vi "IMU Correction.vi"(6 "Enable IMU":bool, 8 "Current Angle":dbl, 9 "Desired Angle (Relative)":dbl, 10 "Iterations":dbl, 11 "PID gains":T1 {"derivative time (Td, min)" format="%.3f"; "integral time (Ti, min)" format="%.3f"; "proportional gain (Kc)" format="%.3f"}) -> (1 "IMU Correction":dbl format="%.2f", 3 "Desired Angle (Absolute)":dbl)   [LabVIEW 2019]
uses:
  <vilib>/addons/control/pid/pid.llb/PID (DBL).vi
  <vilib>/addons/control/pid/NI_PID_pid.lvlib
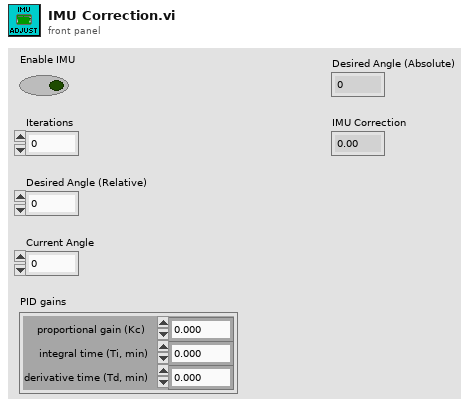
[diagram p1: front panel]
types:
  T1 = cluster{"proportional gain (Kc)":dbl, "integral time (Ti, min)":dbl, "derivative time (Td, min)":dbl}
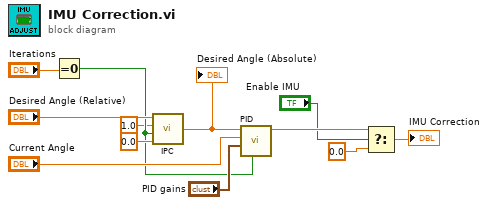
[diagram p0: block diagram]
diagram:
  n1 = Equal To 0?(x="Iterations") -> (x = 0?=w2:bool)
  n2 = call "IPC.vi"("Initilization"=0.0, "Reset"=w2, "Multiplier"=1.0, "Value"="Desired Angle (Relative)") -> ("IPCed"=w8:dbl)  [unwired: 2 in]
  "Desired Angle (Absolute)" <- w8
  n3 = call-poly <vilib>:"PID.vi"("reinitialize? (F)"=w2, "PID gains"="PID gains", "process variable"="Current Angle", "setpoint"=w8) -> ("output"=w6:dbl)  [unwired: 6 in, 1 out]
  n4 = Select(t=w6, s="Enable IMU", f=0.0) -> (s? t:f=→"IMU Correction":dbl)
